vi "AB_900_1000_Project_Build_Info.vi"(7 "action":T1, 8 "error in (no error)":errorcluster, 10 "buildInfo in":T2, 11 "Object In":T3) -> (0 "error out":errorcluster, 2 "buildInfo out":T2, 3 "Object Out":T3)   [LabVIEW 2020]
uses:
  <resource>/Framework/Providers/API/ItemRef.ctl
  <vilib>/AppBuilder/RW_Project/AB_RW_Project_PropBag_Action.ctl
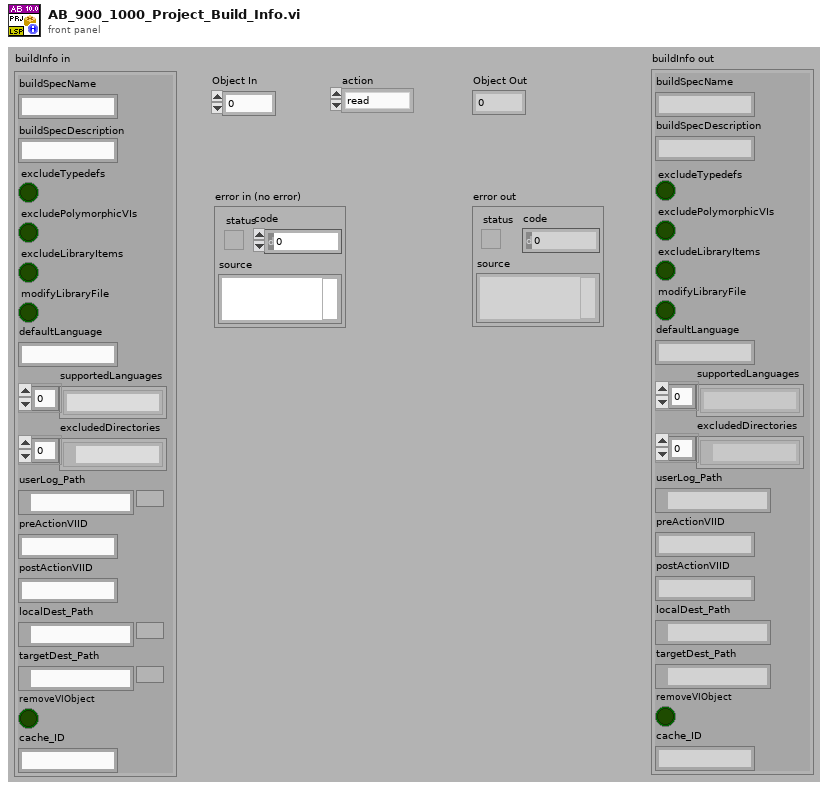
[diagram p1: front panel]
types:
  T1 = typedef "AB_RW_Project_PropBag_Action.ctl" = enum16{"read", "write", "clear", "readPrevious", "writePrevious", "clearPrevious"}
  T2 = cluster{"buildSpecName":string, "buildSpecDescription":string, "excludeTypedefs":bool, "excludePolymorphicVIs":bool, "excludeLibraryItems":bool, "modifyLibraryFile":bool, "defaultLanguage":string, "supportedLanguages":string[], "excludedDirectories":path[], "userLog_Path":path, "preActionVIID":string, "postActionVIID":string, "localDest_Path":path, "targetDest_Path":path, "removeVIObject":bool, "cache_ID":string}
  T3 = typedef "ItemRef.ctl" = u64
  T4 = enum16{"<none>", "relativeToCommon", "relativeToAppDir"}
  T5 = typedef "AB_820_850_Relative_Path_Type.ctl" = enum16{"<none>", "relativeToCommon", "relativeToAppDir"}
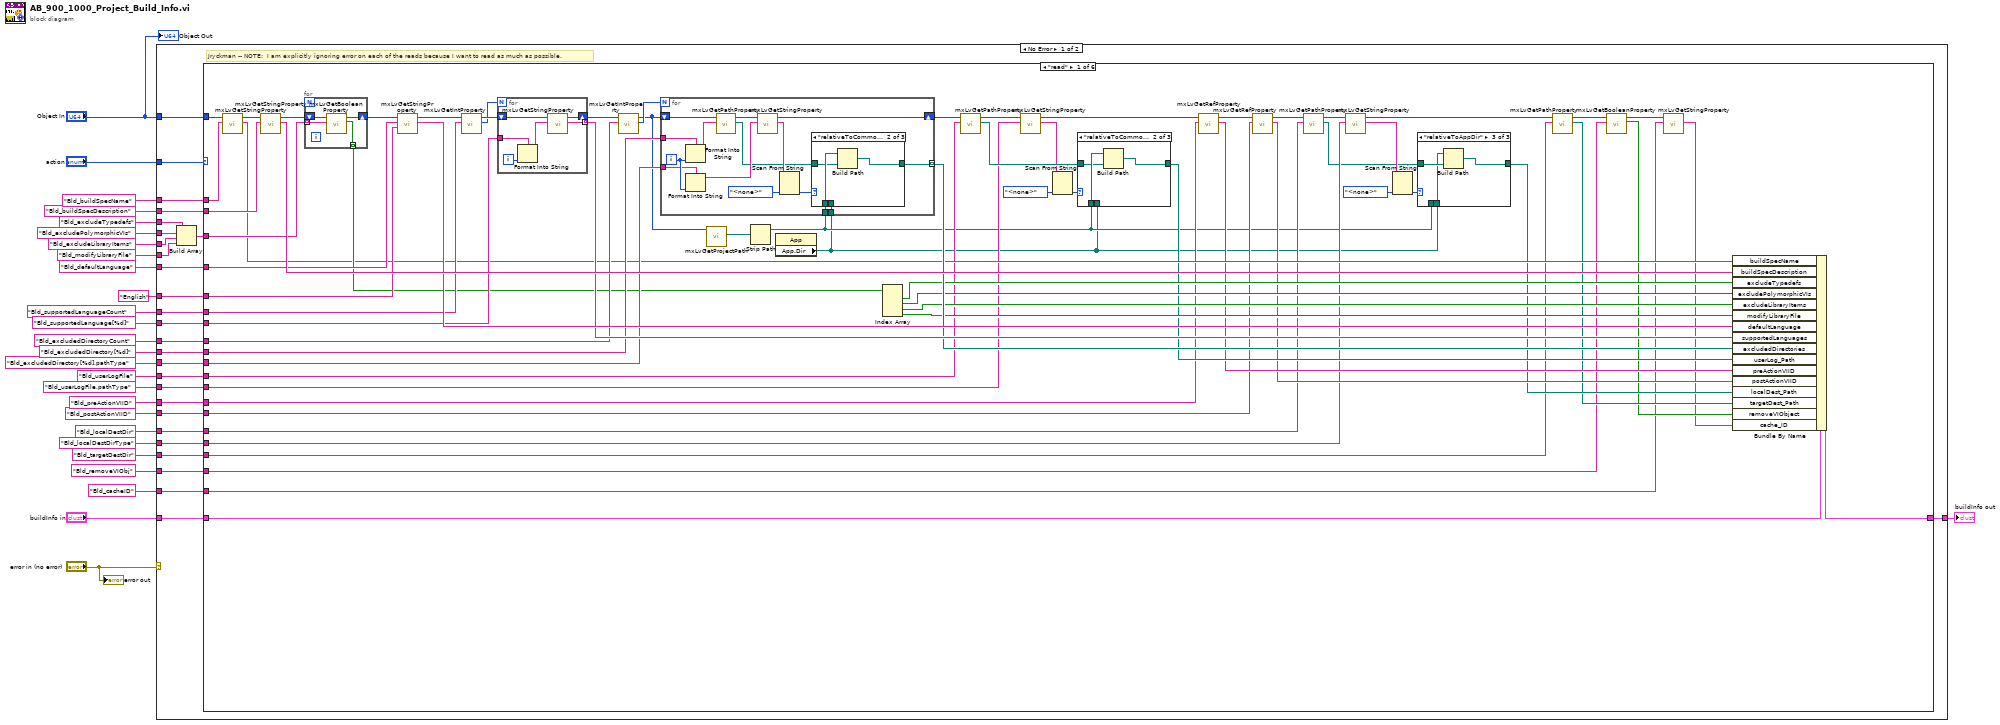
[diagram p0: block diagram]
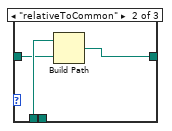
[diagram p3: hidden frame]
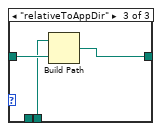
[diagram p5: hidden frame]
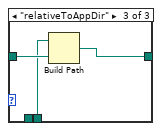
[diagram p7: hidden frame]
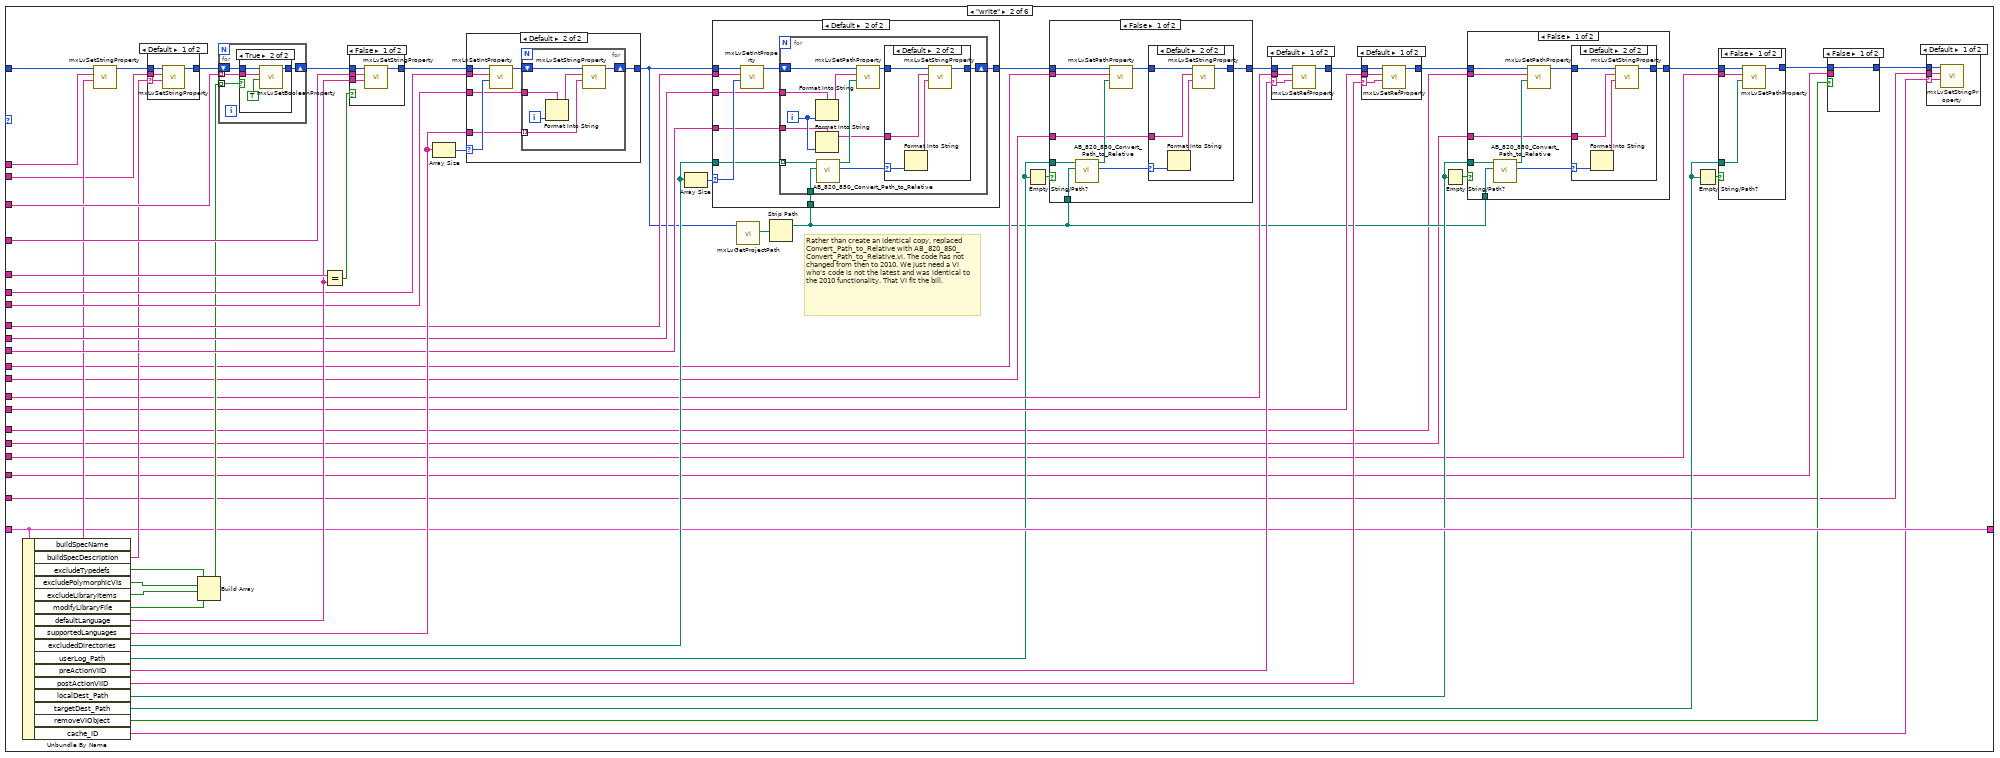
[diagram p8: hidden frame]
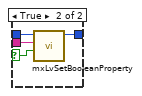
[diagram p10: hidden frame]
diagram:
  n1 = case shown="No Error" "error in (no error)" {
    tunnel: "Object In" -> [w54 _]
    tunnel: [w43 _] -> w25
    tunnel: "Bld_buildSpecDescription" ("Tag") -> [w53 _]
    tunnel: "Bld_excludeTypedefs" ("Tag") -> [w39 _]
    tunnel: "Bld_defaultLanguage" ("Tag") -> [w52 _]
    tunnel: "English" ("Tag") -> [w51 _]
    tunnel: "Bld_supportedLanguageCount" ("Tag") -> [w50 _]
    tunnel: "Bld_supportedLanguage[%d]" ("Tag") -> [w49 _]
    tunnel: "Bld_excludedDirectoryCount" ("Tag") -> [w48 _]
    tunnel: "Bld_excludedDirectory[%d]" ("Tag") -> [w47 _]
    tunnel: "Bld_excludedDirectory[%d].pathType" ("Tag") -> [w46 _]
    tunnel: "buildInfo in" -> [w45 _]
    tunnel: "action" -> [w44 _]
    tunnel: "Bld_excludePolymorphicVIs" ("Tag") -> [w42 _]
    tunnel: "Bld_excludeLibraryItems" ("Tag") -> [w41 _]
    tunnel: "Bld_modifyLibraryFile" ("Tag") -> [w40 _]
    tunnel: "Bld_buildSpecName" ("Tag") -> [w37 _]
    tunnel: "Bld_userLogFile" ("Tag") -> [w36 _]
    tunnel: "Bld_userLogFile.pathType" ("Tag") -> [w35 _]
    tunnel: "Bld_preActionVIID" ("Tag") -> [w34 _]
    tunnel: "Bld_postActionVIID" ("Tag") -> [w33 _]
    tunnel: "Bld_localDestDir" ("Tag") -> [w32 _]
    tunnel: "Bld_targetDestDir" ("Tag") -> [w31 _]
    tunnel: "Bld_localDestDirType" ("Tag") -> [w30 _]
    tunnel: "Bld_removeVIObj" ("Tag") -> [w29 _]
    tunnel: "Bld_cacheID" ("Tag") -> [w28 _]
    frame No Error {
      # "Jryckman -- NOTE:  I am explicitly ignoring error on each of the reads because I want to read as much as possible."
      n2 = Build Array(w39, w42, w41, w40) -> (w38:string[])
      n3 = case shown="\"read\"" w44 {
        tunnel: w54 -> [w95 w205 w376 _ w404 _]
        tunnel: w53 -> [w122 w200 w378 _ _ _]
        tunnel: w52 -> [w120 w225 w377 _ _ _]
        tunnel: w51 -> [w119 w224 _ _ _ _]
        tunnel: w50 -> [w116 w219 w375 _ _ _]
        tunnel: w49 -> [w113 w218 w372 _ _ _]
        tunnel: w48 -> [w110 w214 w368 _ _ _]
        tunnel: w47 -> [w108 w213 w367 _ _ _]
        tunnel: w46 -> [w107 w212 w366 _ _ _]
        tunnel: w45 -> [w104 w184 w363 w395 w408 w409]
        tunnel: [w105 w184 w363 w395 w408 w409] -> w43
        tunnel: w38 -> [w101 w206 w362 _ _ _]
        tunnel: w37 -> [w93 w203 w361 _ _ _]
        tunnel: w36 -> [w88 w197 w359 _ _ _]
        tunnel: w35 -> [w81 w193 w357 _ _ _]
        tunnel: w34 -> [w80 w191 w354 _ w406 _]
        tunnel: w33 -> [w77 w188 w353 _ w405 _]
        tunnel: w32 -> [w69 w179 w350 _ w403 _]
        tunnel: w31 -> [w62 w177 w348 _ w402 _]
        tunnel: w30 -> [w68 w180 w349 _ w400 _]
        tunnel: w29 -> [w58 w173 w345 _ w396 _]
        tunnel: w28 -> [w56 w170 w343 _ _ _]
        frame "read" {
          n4 = call <resource>:"mxLvGetStringProperty.vi"("Tag"=w93, "Item"=w95) -> ("Value"=w92:string, "Item"=w94:T3)  [unwired: 1 in, 7 out]
          n5 = call <resource>:"mxLvGetStringProperty.vi"("Tag"=w122, "Item"=w94) -> ("Value"=w121:string, "Item"=w103:T3)  [unwired: 1 in, 7 out]
          n6 = for {
            shift-right: [w140] -> w102
            shift-left: w103 -> [w138]
            tunnel: w101 -> [w139] mode=indexing
            tunnel: [w137] -> w100 mode=indexing
            n7 = call <resource>:"mxLvGetBooleanProperty.vi"("Tag"=w139, "Item"=w138) -> ("Value"=w137:bool, "Item"=w140:T3)  [unwired: 1 in, 7 out]
          }
          n8 = call <resource>:"mxLvGetStringProperty.vi"("Default Value (\"\")"=w119, "Tag"=w120, "Item"=w102) -> ("Value"=w118:string, "Item"=w117:T3)  [unwired: 1 in, 6 out]
          n9 = call <resource>:"mxLvGetIntProperty.vi"("Tag"=w116, "Item"=w117) -> ("Value"=w114:i32, "Item"=w115:T3)  [unwired: 1 in, 7 out]
          n10 = for {
            N: w114 -> [_]
            shift-right: [w165] -> w111
            shift-left: w115 -> [w166]
            tunnel: w113 -> [w167]
            tunnel: [w163] -> w112 mode=indexing
            i -> [w168]
            n11 = Format Into String(format string=w167, w168) -> (resulting string=w164:string)  [unwired: 2 in, 1 out]
            n12 = call <resource>:"mxLvGetStringProperty.vi"("Tag"=w164, "Item"=w166) -> ("Value"=w163:string, "Item"=w165:T3)  [unwired: 1 in, 7 out]
          }
          n13 = call <resource>:"mxLvGetIntProperty.vi"("Tag"=w110, "Item"=w111) -> ("Value"=w109:i32, "Item"=w91:T3)  [unwired: 1 in, 7 out]
          n14 = call <resource>:"mxLvGetProjectPath.vi"("Item"=w91) -> ("Project Path"=w90:path)  [unwired: 1 in, 9 out]
          n15 = Strip Path(path=w90) -> (stripped path=w66:path)  [unwired: 1 out]
          n16 = property class="App"() -> ("App.Dir"=w65:path)  [unwired: 2 in, 2 out]
          n17 = for {
            N: w109 -> [_]
            shift-right: [w142] -> w89
            shift-left: w91 -> [w152]
            tunnel: w108 -> [w155]
            tunnel: w107 -> [w153]
            tunnel: w66 -> [w145]
            tunnel: [w143] -> w106 mode=indexing
            tunnel: w65 -> [w141]
            i -> [w154]
            n18 = Format Into String(format string=w155, w154) -> (resulting string=w151:string)  [unwired: 2 in, 1 out]
            n19 = Format Into String(format string=w153, w154) -> (resulting string=w149:string)  [unwired: 2 in, 1 out]
            n20 = call <resource>:"mxLvGetPathProperty.vi"("Tag"=w151, "Item"=w152) -> ("Path"=w144:path, "Item"=w150:T3)  [unwired: 2 in, 6 out]
            n21 = call <resource>:"mxLvGetStringProperty.vi"("Tag"=w149, "Item"=w150) -> ("Value"=w148:string, "Item"=w142:T3)  [unwired: 1 in, 7 out]
            n22 = Scan From String(input string=w148, default 1=T4."<none>" ("relativeType")) -> (output 1=w146:T4)  [unwired: 3 in, 3 out]
            n23 = case shown="\"relativeToCommon\"" w146 {
              tunnel: w145 -> [_ w159 _]
              tunnel: w144 -> [w156 w158 w162]
              tunnel: [w156 w157 w161] -> w143
              tunnel: w141 -> [_ _ w160]
              frame "<none>" {
              }
              frame "relativeToCommon" {
                n24 = Build Path(base path=w159, name or relative path=w158) -> (appended path=w157:path)
              }
              frame "relativeToAppDir" {
                n25 = Build Path(base path=w160, name or relative path=w162) -> (appended path=w161:path)
              }
            }
          }
          n26 = Index Array(array=w100) -> (element #1=w99:bool, element #2=w98:bool, element #3=w97:bool, element #4=w96:bool)  [unwired: 4 in]
          n27 = call <resource>:"mxLvGetPathProperty.vi"("Tag"=w88, "Item"=w89) -> ("Path"=w85:path, "Item"=w83:T3)  [unwired: 2 in, 6 out]
          n28 = call <resource>:"mxLvGetStringProperty.vi"("Tag"=w81, "Item"=w83) -> ("Value"=w82:string, "Item"=w79:T3)  [unwired: 1 in, 7 out]
          n29 = Scan From String(input string=w82, default 1=T4."<none>" ("relativeType")) -> (output 1=w87:T4)  [unwired: 3 in, 3 out]
          n30 = case shown="\"relativeToCommon\"" w87 {
            tunnel: w66 -> [_ w133 _]
            tunnel: w85 -> [w130 w132 w136]
            tunnel: [w130 w131 w135] -> w84
            tunnel: w65 -> [_ _ w134]
            frame "<none>" {
            }
            frame "relativeToCommon" {
              n31 = Build Path(base path=w133, name or relative path=w132) -> (appended path=w131:path)
            }
            frame "relativeToAppDir" {
              n32 = Build Path(base path=w134, name or relative path=w136) -> (appended path=w135:path)
            }
          }
          n33 = call <resource>:"mxLvGetRefProperty.vi"("Tag"=w80, "Item"=w79) -> ("Value"=w78:string, "Item"=w76:T3)  [unwired: 1 in, 7 out]
          n34 = call <resource>:"mxLvGetRefProperty.vi"("Tag"=w77, "Item"=w76) -> ("Value"=w75:string, "Item"=w70:T3)  [unwired: 1 in, 7 out]
          n35 = call <resource>:"mxLvGetPathProperty.vi"("Tag"=w69, "Item"=w70) -> ("Path"=w67:path, "Item"=w71:T3)  [unwired: 2 in, 6 out]
          n36 = call <resource>:"mxLvGetStringProperty.vi"("Tag"=w68, "Item"=w71) -> ("Value"=w74:string, "Item"=w63:T3)  [unwired: 1 in, 7 out]
          n37 = Scan From String(input string=w74, default 1=T4."<none>" ("relativeType")) -> (output 1=w72:T4)  [unwired: 3 in, 3 out]
          n38 = case shown="\"relativeToAppDir\"" w72 {
            tunnel: w66 -> [_ w126 _]
            tunnel: w67 -> [w123 w125 w129]
            tunnel: [w123 w124 w128] -> w64
            tunnel: w65 -> [_ _ w127]
            frame "<none>" {
            }
            frame "relativeToCommon" {
              n39 = Build Path(base path=w126, name or relative path=w125) -> (appended path=w124:path)
            }
            frame "relativeToAppDir" {
              n40 = Build Path(base path=w127, name or relative path=w129) -> (appended path=w128:path)
            }
          }
          n41 = call <resource>:"mxLvGetPathProperty.vi"("Tag"=w62, "Item"=w63) -> ("Path"=w61:path, "Item"=w60:T3)  [unwired: 2 in, 6 out]
          n42 = call <resource>:"mxLvGetBooleanProperty.vi"("Tag"=w58, "Item"=w60) -> ("Value"=w59:bool, "Item"=w57:T3)  [unwired: 1 in, 7 out]
          n43 = call <resource>:"mxLvGetStringProperty.vi"("Tag"=w56, "Item"=w57) -> ("Value"=w55:string)  [unwired: 1 in, 8 out]
          n44 = Bundle By Name(cluster=w104, "buildSpecName"=w92, "buildSpecDescription"=w121, "excludeTypedefs"=w99, "excludePolymorphicVIs"=w98, "excludeLibraryItems"=w97, "modifyLibraryFile"=w96, "defaultLanguage"=w118, "supportedLanguages"=w112, "excludedDirectories"=w106, "userLog_Path"=w84, "preActionVIID"=w78, "postActionVIID"=w75, "localDest_Path"=w64, "targetDest_Path"=w61, "removeVIObject"=w59, "cache_ID"=w55) -> (w105:T2)
        }
        frame "write" {
          # "Rather than create an identical copy, replaced  Convert_Path_to_Relative with AB_820_850_Convert_Path_to_Relative.vi. The code has not changed from then to 2010. We just need a VI who's code is not the latest and was identical to the 2010 functionality. That VI fit the bill."
          n45 = Unbundle By Name(w184) -> ("buildSpecName"=w204:string, "buildSpecDescription"=w199:string, "excludeTypedefs"=w211:bool, "excludePolymorphicVIs"=w210:bool, "excludeLibraryItems"=w209:bool, "modifyLibraryFile"=w208:bool, "defaultLanguage"=w223:string, "supportedLanguages"=w217:string[], "excludedDirectories"=w215:path[], "userLog_Path"=w183:path, "preActionVIID"=w190:string, "postActionVIID"=w187:string, "localDest_Path"=w182:path, "targetDest_Path"=w176:path, "removeVIObject"=w172:bool, "cache_ID"=w169:string)
          n46 = call <resource>:"mxLvSetStringProperty.vi"("Value (\"\")"=w204, "Tag"=w203, "Item"=w205) -> ("Item"=w202:T3)  [unwired: 2 in, 6 out]
          n47 = case shown="Default" w199 {
            selector: w199 -> [w282 _]
            tunnel: w202 -> [w285 w286]
            tunnel: w200 -> [w284 _]
            tunnel: [w283 w286] -> w201
            frame Default {
              n48 = call <resource>:"mxLvSetStringProperty.vi"("Value (\"\")"=w282, "Tag"=w284, "Item"=w285) -> ("Item"=w283:T3)  [unwired: 2 in, 6 out]
            }
            frame "" {
            }
          }
          n49 = Build Array(w211, w210, w209, w208) -> (w207:bool[])
          n50 = for {
            shift-right: [w289] -> w226
            shift-left: w201 -> [w290]
            tunnel: w207 -> [w288] mode=indexing
            tunnel: w206 -> [w287] mode=indexing
            n51 = case shown="True" w288 {
              tunnel: w290 -> [w291 w295]
              tunnel: [w291 w294] -> w289
              tunnel: w287 -> [_ w293]
              frame False {
              }
              frame True {
                n52 = call <resource>:"mxLvSetBooleanProperty.vi"("Value (F)"=TRUE, "Tag"=w293, "Item"=w295) -> ("Item"=w294:T3)  [unwired: 2 in, 6 out]
              }
            }
          }
          n53 = Equal?(x=w224, y=w223) -> (x = y?=w222:bool)
          n54 = case shown="False" w222 {
            tunnel: w226 -> [w341 w342]
            tunnel: w225 -> [w340 _]
            tunnel: w223 -> [w339 _]
            tunnel: [w338 w342] -> w220
            frame False {
              n55 = call <resource>:"mxLvSetStringProperty.vi"("Value (\"\")"=w339, "Tag"=w340, "Item"=w341) -> ("Item"=w338:T3)  [unwired: 2 in, 6 out]
            }
            frame True {
            }
          }
          n56 = Array Size(array=w217) -> (size(s)=w221:i32)
          n57 = case shown="Default" w221 {
            selector: w221 -> [_ w329]
            tunnel: w220 -> [w324 w331]
            tunnel: w219 -> [_ w330]
            tunnel: w218 -> [_ w327]
            tunnel: w217 -> [_ w326]
            tunnel: [w324 w325] -> w194
            frame 0 {
            }
            frame Default {
              n58 = call <resource>:"mxLvSetIntProperty.vi"("Value (0)"=w329, "Tag"=w330, "Item"=w331) -> ("Item"=w328:T3)  [unwired: 2 in, 6 out]
              n59 = for {
                shift-right: [w336] -> w325
                shift-left: w328 -> [w337]
                tunnel: w327 -> [w334]
                tunnel: w326 -> [w332] mode=indexing
                i -> [w335]
                n60 = Format Into String(format string=w334, w335) -> (resulting string=w333:string)  [unwired: 2 in, 1 out]
                n61 = call <resource>:"mxLvSetStringProperty.vi"("Value (\"\")"=w332, "Tag"=w333, "Item"=w337) -> ("Item"=w336:T3)  [unwired: 2 in, 6 out]
              }
            }
          }
          n62 = Array Size(array=w215) -> (size(s)=w216:i32)
          n63 = call <resource>:"mxLvGetProjectPath.vi"("Item"=w194) -> ("Project Path"=w195:path)  [unwired: 1 in, 9 out]
          n64 = Strip Path(path=w195) -> (stripped path=w181:path)  [unwired: 1 out]
          n65 = case shown="Default" w216 {
            selector: w216 -> [_ w304]
            tunnel: w194 -> [w296 w299]
            tunnel: w214 -> [_ w305]
            tunnel: w213 -> [_ w302]
            tunnel: w215 -> [_ w301]
            tunnel: w212 -> [_ w300]
            tunnel: [w296 w298] -> w198
            tunnel: w181 -> [_ w297]
            frame 0 {
            }
            frame Default {
              n66 = call <resource>:"mxLvSetIntProperty.vi"("Value (0)"=w304, "Tag"=w305, "Item"=w299) -> ("Item"=w303:T3)  [unwired: 2 in, 6 out]
              n67 = for {
                shift-right: [w317] -> w298
                shift-left: w303 -> [w313]
                tunnel: w302 -> [w316]
                tunnel: w301 -> [w315] mode=indexing
                tunnel: w297 -> [w307]
                tunnel: w300 -> [w306]
                i -> [w311]
                n68 = Format Into String(format string=w316, w311) -> (resulting string=w314:string)  [unwired: 2 in, 1 out]
                n69 = Format Into String(format string=w306, w311) -> (resulting string=w309:string)  [unwired: 2 in, 1 out]
                n70 = call <vilib>:"AB_820_850_Convert_Path_to_Relative.vi"("commonPath"=w307, "absolutePath"=w315) -> ("relativeType"=w308:T5, "newPath"=w310:path)  [unwired: 7 in, 1 out]
                n71 = call <resource>:"mxLvSetPathProperty.vi"("Path"=w310, "Tag"=w314, "Item"=w313) -> ("Item"=w312:T3)  [unwired: 2 in, 6 out]
                n72 = case shown="Default" w308 {
                  selector: w308 -> [_ w319]
                  tunnel: [w318 w323] -> w317
                  tunnel: w312 -> [w318 w322]
                  tunnel: w309 -> [_ w320]
                  frame "<none>" {
                  }
                  frame Default {
                    n73 = Format Into String(w319) -> (resulting string=w321:string)  [unwired: 3 in, 1 out]
                    n74 = call <resource>:"mxLvSetStringProperty.vi"("Value (\"\")"=w321, "Tag"=w320, "Item"=w322) -> ("Item"=w323:T3)  [unwired: 2 in, 6 out]
                  }
                }
              }
            }
          }
          n75 = Empty String/Path?(string/path=w183) -> (empty?=w196:bool)
          n76 = case shown="False" w196 {
            tunnel: w198 -> [w274 w281]
            tunnel: w197 -> [w273 _]
            tunnel: w181 -> [w270 _]
            tunnel: w183 -> [w269 _]
            tunnel: w193 -> [w267 _]
            tunnel: [w266 w281] -> w192
            frame False {
              n77 = call <vilib>:"AB_820_850_Convert_Path_to_Relative.vi"("commonPath"=w270, "absolutePath"=w269) -> ("relativeType"=w272:T5, "newPath"=w268:path)  [unwired: 7 in, 1 out]
              n78 = call <resource>:"mxLvSetPathProperty.vi"("Path"=w268, "Tag"=w273, "Item"=w274) -> ("Item"=w271:T3)  [unwired: 2 in, 6 out]
              n79 = case shown="Default" w272 {
                selector: w272 -> [_ w277]
                tunnel: w271 -> [w275 w280]
                tunnel: w267 -> [_ w278]
                tunnel: [w275 w276] -> w266
                frame "<none>" {
                }
                frame Default {
                  n80 = Format Into String(w277) -> (resulting string=w279:string)  [unwired: 3 in, 1 out]
                  n81 = call <resource>:"mxLvSetStringProperty.vi"("Value (\"\")"=w279, "Tag"=w278, "Item"=w280) -> ("Item"=w276:T3)  [unwired: 2 in, 6 out]
                }
              }
            }
            frame True {
            }
          }
          n82 = case shown="Default" w190 {
            selector: w190 -> [w262 _]
            tunnel: w192 -> [w264 w265]
            tunnel: w191 -> [w263 _]
            tunnel: [w261 w265] -> w189
            frame Default {
              n83 = call <resource>:"mxLvSetRefProperty.vi"("Value (\"\")"=w262, "Tag"=w263, "Item"=w264) -> ("Item"=w261:T3)  [unwired: 2 in, 6 out]
            }
            frame "" {
            }
          }
          n84 = case shown="Default" w187 {
            selector: w187 -> [w257 _]
            tunnel: w189 -> [w259 w260]
            tunnel: w188 -> [w258 _]
            tunnel: [w256 w260] -> w185
            frame Default {
              n85 = call <resource>:"mxLvSetRefProperty.vi"("Value (\"\")"=w257, "Tag"=w258, "Item"=w259) -> ("Item"=w256:T3)  [unwired: 2 in, 6 out]
            }
            frame "" {
            }
          }
          n86 = Empty String/Path?(string/path=w182) -> (empty?=w186:bool)
          n87 = case shown="False" w186 {
            tunnel: w185 -> [w248 w255]
            tunnel: w179 -> [w247 _]
            tunnel: w181 -> [w244 _]
            tunnel: w182 -> [w243 _]
            tunnel: w180 -> [w241 _]
            tunnel: [w240 w255] -> w178
            frame False {
              n88 = call <vilib>:"AB_820_850_Convert_Path_to_Relative.vi"("commonPath"=w244, "absolutePath"=w243) -> ("relativeType"=w246:T5, "newPath"=w242:path)  [unwired: 7 in, 1 out]
              n89 = call <resource>:"mxLvSetPathProperty.vi"("Path"=w242, "Tag"=w247, "Item"=w248) -> ("Item"=w245:T3)  [unwired: 2 in, 6 out]
              n90 = case shown="Default" w246 {
                selector: w246 -> [_ w251]
                tunnel: w245 -> [w249 w254]
                tunnel: w241 -> [_ w252]
                tunnel: [w249 w250] -> w240
                frame "<none>" {
                }
                frame Default {
                  n91 = Format Into String(w251) -> (resulting string=w253:string)  [unwired: 3 in, 1 out]
                  n92 = call <resource>:"mxLvSetStringProperty.vi"("Value (\"\")"=w253, "Tag"=w252, "Item"=w254) -> ("Item"=w250:T3)  [unwired: 2 in, 6 out]
                }
              }
            }
            frame True {
            }
          }
          n93 = Empty String/Path?(string/path=w176) -> (empty?=w175:bool)
          n94 = case shown="False" w175 {
            tunnel: w178 -> [w238 w239]
            tunnel: w177 -> [w237 _]
            tunnel: w176 -> [w236 _]
            tunnel: [w235 w239] -> w174
            frame False {
              n95 = call <resource>:"mxLvSetPathProperty.vi"("Path"=w236, "Tag"=w237, "Item"=w238) -> ("Item"=w235:T3)  [unwired: 2 in, 6 out]
            }
            frame True {
            }
          }
          n96 = case shown="False" w172 {
            selector: w172 -> [_ w232]
            tunnel: w174 -> [w230 w234]
            tunnel: w173 -> [_ w233]
            tunnel: [w230 w231] -> w171
            frame False {
            }
            frame True {
              n97 = call <resource>:"mxLvSetBooleanProperty.vi"("Value (F)"=w232, "Tag"=w233, "Item"=w234) -> ("Item"=w231:T3)  [unwired: 2 in, 6 out]
            }
          }
          n98 = case shown="Default" w169 {
            selector: w169 -> [w227 _]
            tunnel: w171 -> [w229 _]
            tunnel: w170 -> [w228 _]
            frame Default {
              n99 = call <resource>:"mxLvSetStringProperty.vi"("Value (\"\")"=w227, "Tag"=w228, "Item"=w229) -> ()  [unwired: 2 in, 7 out]
            }
            frame "" {
            }
          }
        }
        frame "clear" {
          n100 = Build Array (concatenate)(w361, w378, w362, w377, w375, w368) -> (w364:string[])
          n101 = call <resource>:"mxLvGetIntProperty.vi"("Tag"=w375, "Item"=w376) -> ("Value"=w373:i32, "Item"=w374:T3)  [unwired: 1 in, 7 out]
          n102 = for {
            N: w373 -> [_]
            shift-right: [w391] -> w369
            shift-left: w374 -> [w392]
            tunnel: w372 -> [w393]
            i -> [w394]
            n103 = Format Into String(format string=w393, w394) -> (resulting string=w390:string)  [unwired: 2 in, 1 out]
            n104 = call <resource>:"mxLvDeleteProperty.vi"("Tag"=w390, "Item"=w392) -> ("Item"=w391:T3)  [unwired: 1 in, 8 out]
          }
          n105 = call <resource>:"mxLvGetIntProperty.vi"("Tag"=w368, "Item"=w369) -> ("Value"=w371:i32, "Item"=w370:T3)  [unwired: 1 in, 7 out]
          n106 = for {
            N: w371 -> [_]
            shift-right: [w385] -> w365
            shift-left: w370 -> [w388]
            tunnel: w367 -> [w389]
            tunnel: w366 -> [w383]
            i -> [w384]
            n107 = Format Into String(format string=w389, w384) -> (resulting string=w387:string)  [unwired: 2 in, 1 out]
            n108 = Format Into String(format string=w383, w384) -> (resulting string=w382:string)  [unwired: 2 in, 1 out]
            n109 = call <resource>:"mxLvDeleteProperty.vi"("Tag"=w387, "Item"=w388) -> ("Item"=w386:T3)  [unwired: 1 in, 8 out]
            n110 = call <resource>:"mxLvDeleteProperty.vi"("Tag"=w382, "Item"=w386) -> ("Item"=w385:T3)  [unwired: 1 in, 8 out]
          }
          n111 = for {
            tunnel: w364 -> [w380] mode=indexing
            shift-right: [w379] -> w360
            shift-left: w365 -> [w381]
            n112 = call <resource>:"mxLvDeleteProperty.vi"("Tag"=w380, "Item"=w381) -> ("Item"=w379:T3)  [unwired: 1 in, 8 out]
          }
          n113 = call <resource>:"mxLvDeleteProperty.vi"("Tag"=w359, "Item"=w360) -> ("Item"=w358:T3)  [unwired: 1 in, 8 out]
          n114 = call <resource>:"mxLvDeleteProperty.vi"("Tag"=w357, "Item"=w358) -> ("Item"=w355:T3)  [unwired: 1 in, 8 out]
          n115 = call <resource>:"mxLvDeleteProperty.vi"("Tag"=w354, "Item"=w355) -> ("Item"=w356:T3)  [unwired: 1 in, 8 out]
          n116 = call <resource>:"mxLvDeleteProperty.vi"("Tag"=w353, "Item"=w356) -> ("Item"=w347:T3)  [unwired: 1 in, 8 out]
          n117 = call <resource>:"mxLvDeleteProperty.vi"("Tag"=w350, "Item"=w347) -> ("Item"=w352:T3)  [unwired: 1 in, 8 out]
          n118 = call <resource>:"mxLvDeleteProperty.vi"("Tag"=w349, "Item"=w352) -> ("Item"=w351:T3)  [unwired: 1 in, 8 out]
          n119 = call <resource>:"mxLvDeleteProperty.vi"("Tag"=w348, "Item"=w351) -> ("Item"=w346:T3)  [unwired: 1 in, 8 out]
          n120 = call <resource>:"mxLvDeleteProperty.vi"("Tag"=w345, "Item"=w346) -> ("Item"=w344:T3)  [unwired: 1 in, 8 out]
          n121 = call <resource>:"mxLvDeleteProperty.vi"("Tag"=w343, "Item"=w344) -> ()  [unwired: 1 in, 9 out]
        }
        frame "readPrevious" {
        }
        frame "writePrevious" {
          n122 = call <resource>:"mxLvDeleteProperty.vi"("Tag"=w406, "Item"=w404) -> ("Item"=w407:T3)  [unwired: 1 in, 8 out]
          n123 = call <resource>:"mxLvDeleteProperty.vi"("Tag"=w405, "Item"=w407) -> ("Item"=w401:T3)  [unwired: 1 in, 8 out]
          n124 = call <resource>:"mxLvDeleteProperty.vi"("Tag"=w403, "Item"=w401) -> ("Item"=w399:T3)  [unwired: 1 in, 8 out]
          n125 = call <resource>:"mxLvDeleteProperty.vi"("Tag"=w400, "Item"=w399) -> ("Item"=w398:T3)  [unwired: 1 in, 8 out]
          n126 = call <resource>:"mxLvDeleteProperty.vi"("Tag"=w402, "Item"=w398) -> ("Item"=w397:T3)  [unwired: 1 in, 8 out]
          n127 = call <resource>:"mxLvDeleteProperty.vi"("Tag"=w396, "Item"=w397) -> ()  [unwired: 1 in, 9 out]
        }
        frame "clearPrevious" {
        }
      }
    }
    frame Error {
    }
  }
  "buildInfo out" <- w25
  "Object Out" <- "Object In"
  "error out" <- "error in (no error)"
